vi "VI Tree.vi"   [LabVIEW 2020, in "RIGOL DP1000 Series.lvlib"]
doc: "This is the instrument driver for the RIGOL DP1000 Series. The VI Tree displays all the user-callable VIs of the instrument driver in an organized table."
uses:
  <instrlib>/RIGOL DP1000 Series/RIGOL DP1000 Series.lvlib
panel:
  # "(c) 2011-2012 National Instruments.  ALL RIGHTS RESERVED."
  # "SEE DIAGRAM\nFOR VI TREE."
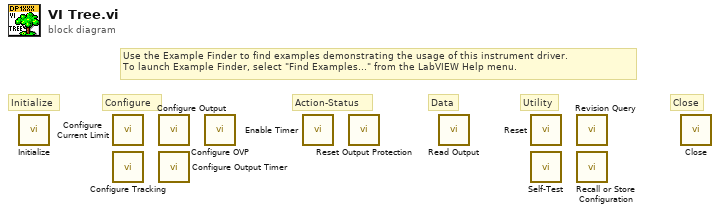
[diagram p0: block diagram]
diagram:
  # "Close"
  # "Utility"
  # "Data"
  # "Configure"
  # "Action-Status"
  # "Initialize"
  # "Use the Example Finder to find examples demonstrating the usage of this instrument driver.\nTo launch Example Finder, select \"Find Examples...\" from the LabVIEW Help menu."
  n1 = call <instrlib>:"Initialize.vi"() -> ()  [unwired: 10 in, 2 out]
  n2 = call <instrlib>:"Configure Current Limit.vi"() -> ()  [unwired: 10 in, 2 out]
  n3 = call <instrlib>:"Configure Tracking.vi"() -> ()  [unwired: 10 in, 2 out]
  n4 = call <instrlib>:"Configure Output.vi"() -> ()  [unwired: 10 in, 2 out]
  n5 = call <instrlib>:"Configure Output Timer.vi"() -> ()  [unwired: 10 in, 2 out]
  n6 = call <instrlib>:"Configure OVP.vi"() -> ()  [unwired: 10 in, 2 out]
  n7 = call <instrlib>:"Enable Timer.vi"() -> ()  [unwired: 10 in, 2 out]
  n8 = call <instrlib>:"Reset Output Protection.vi"() -> ()  [unwired: 10 in, 2 out]
  n9 = call <instrlib>:"Read Output.vi"() -> ()  [unwired: 7 in, 5 out]
  n10 = call <instrlib>:"Reset.vi"() -> ()  [unwired: 10 in, 2 out]
  n11 = call <instrlib>:"Self-Test.vi"() -> ()  [unwired: 8 in, 4 out]
  n12 = call <instrlib>:"Revision Query.vi"() -> ()  [unwired: 8 in, 4 out]
  n13 = call <instrlib>:"Recall or Store Configuration.vi"() -> ()  [unwired: 10 in, 2 out]
  n14 = call <instrlib>:"Close.vi"() -> ()  [unwired: 11 in, 1 out]
